vi "init.vi"(8 "error in":errorcluster, 10 "TBM module configuration in":refnum<class "TBM module configuration.lvclass">, 11 "UI Reference runtime in":refnum<class "UI Reference runtime.lvclass">) -> (0 "error out":errorcluster, 1 "data allocations":T1, 2 "execution settings":T4, 3 "UI Reference runtime out":refnum<class "UI Reference runtime.lvclass">)   [LabVIEW 2015, in "UI Reference runtime.lvclass"]
doc: "Provides an interface for initializing a module at runtime. While this interface performs no operations, a child should provide an override which may open any necessary references or sessions, allocate necessary memory, and perform any final configuration validataion before providing the full configuration <b>execution data</b> to the calling process."
uses:
  UI Reference runtime.lvclass
  <vilib>/NI/Tag Bus Module Framework/module configuration/TBM module configuration.lvclass
  <vilib>/NI/Tag Bus Module Framework/runtime/execution settings.ctl
  <vilib>/NI/Tag Bus Module Framework/channel/data tables.ctl
  <vilib>/NI/Tag Bus/dictionary/data dictionary.lvclass
  <vilib>/NI/Tag Bus/dictionary table pair.ctl
  <vilib>/NI/Tag Bus/table/data table.ctl
  configuration/UI Reference configuration.lvclass
  UI Reference runtime.lvclass/UI Reference runtime.ctl
  <vilib>/NI/Tag Bus Module Framework/channel/TBM channel.lvclass
  <vilib>/NI/Tag Bus Module Framework/runtime/TBM module execution interface.lvclass
  <vilib>/NI/Tag Bus/tag bus.lvlib
  <vilib>/NI/Tag Bus/table/data table.lvlib
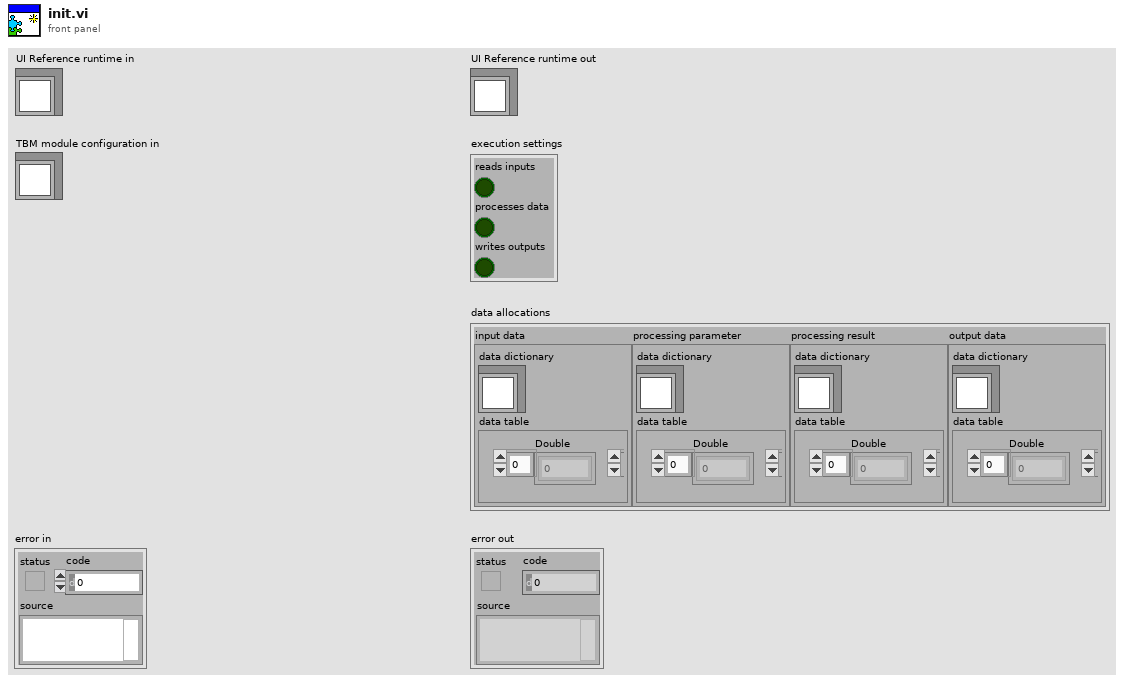
[diagram p1: front panel]
types:
  T1 = typedef "TBM channel.lvclass/data tables.ctl" = cluster{"input data":T2, "processing parameter":T2, "processing result":T2, "output data":T2}
  T2 = typedef "tag bus.lvlib/dictionary table pair.ctl" = cluster{"data dictionary":refnum<class "data dictionary.lvclass">, "data table":T3}
  T3 = typedef "tag bus.lvlib/data table.lvlib/data table.ctl" = cluster{"Double":dbl[], "Single":sgl[], "I64":i64[], "I32":i32[], "I16":i16[], "I8":i8[], "U64":u64[], "U32":u32[], "U16":u16[], "U8":u8[], "Boolean":bool[], "String":string[], "Array of Double":cluster{"DBL Array":dbl[]}[], "Array of Single":cluster{"SGL Array":sgl[]}[], "Array of I64":cluster{"I64 Array":i64[]}[], "Array of I32":cluster{"I32 Array":i32[]}[], "Array of I16":cluster{"I16 Array":i16[]}[], "Array of I8":cluster{"I8 Array":i8[]}[], "Array of U64":cluster{"U64 Array":u64[]}[], "Array of U32":cluster{"U32 Array":u32[]}[], "Array of U16":cluster{"U16 Array":u16[]}[], "Array of U8":cluster{"U8 Array":u8[]}[], "Array of Boolean":cluster{"Boolean Array":bool[]}[], "Array of String":cluster{"String Array":string[]}[]}
  T4 = typedef "TBM module execution interface.lvclass/execution settings.ctl" = cluster{"reads inputs":bool, "processes data":bool, "writes outputs":bool}
  T5 = typedef "UI Reference runtime.lvclass/Mapping.ctl" = cluster{"data type":T6, "control indexes":i32[], "data indexes":i32[]}
  T6 = typedef "tag bus.lvlib/tag descriptor.lvclass/Data Type.ctl" = enum16{"Double", "Single", "I64", "I32", "I16", "I8", "U64", "U32", "U16", "U8", "Boolean", "String", "Array of Double", "Array of Single", "Array of I64", "Array of I32", "Array of I16", "Array of I8", "Array of U64", "Array of U32", "Array of U16", "Array of U8", "Array of Boolean", "Array of String"}
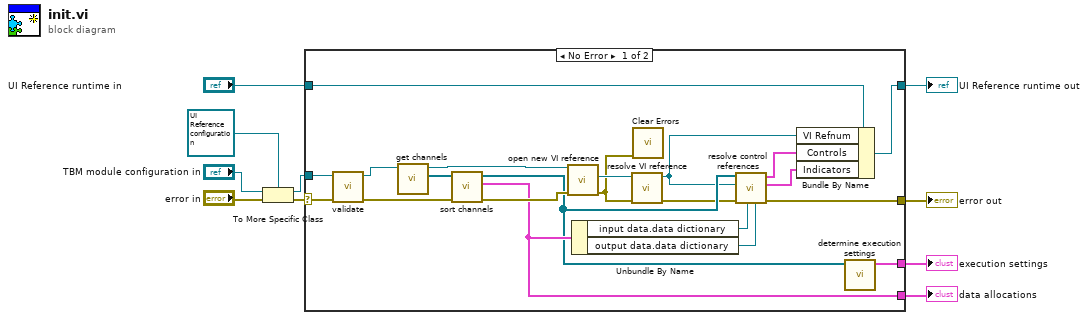
[diagram p0: block diagram]
diagram:
  n1 = To More Specific Class(target class=refnum<class "UI Reference configuration.lvclass"> refnum ("Synchronous module configuration"), reference="TBM module configuration in", error in="error in") -> (specific class reference=w9:refnum<class "UI Reference configuration.lvclass">, error out=w10:errorcluster)
  n2 = case shown="No Error" w10 {
    selector: w10 -> [w29 w32]
    tunnel: w9 -> [w28 _]
    tunnel: "UI Reference runtime in" -> [w17 w33]
    tunnel: [w16 w33] -> w4
    tunnel: [w11 w32] -> w3
    tunnel: [w21 _] -> w1
    tunnel: [w31 _] -> w2
    frame No Error {
      n3 = call-dynamic "validate.vi"("error in"=w29, "UI Reference configuration in"=w28) -> ("error out"=w30:errorcluster, "UI Reference configuration out"=w27:refnum<class "UI Reference configuration.lvclass">)  [unwired: 8 in]
      n4 = call-dynamic "get channels.vi"("UI Reference configuration in"=w27) -> ("channels"=w26:refnum<class "TBM channel.lvclass">[], "UI Reference configuration out"=w25:refnum<class "UI Reference configuration.lvclass">)  [unwired: 9 in]
      n5 = call <vilib>:"sort channels.vi"("error in"=w30, "channels in"=w26) -> ("error out"=w24:errorcluster, "data allocations"=w21:T1, "channels out"=w20:refnum<class "TBM channel.lvclass">[])  [unwired: 7 in]
      n6 = call "open new VI reference.vi"("error in"=w24, "UI Reference configuration in"=w25) -> ("error out"=w22:errorcluster, "VI Refnum"=w23:refnum<vi>)  [unwired: 7 in, 1 out]
      n7 = Unbundle By Name(w21) -> ("input data.data dictionary"=w19:refnum<class "data dictionary.lvclass">, "output data.data dictionary"=w18:refnum<class "data dictionary.lvclass">)
      n8 = call "resolve VI reference.vi"("error in"=w22, "VI reference"=w23) -> ("error out"=w14:errorcluster, "UI Ref"=w15:refnum<vi>)  [unwired: 8 in]
      n9 = call <vilib>:"Clear Errors.vi"("error in (no error)"=w22) -> ()  [unwired: 5 in, 2 out]
      n10 = call "resolve control references.vi"("output dictionary"=w18, "input dictionary"=w19, "error in"=w14, "UI Ref"=w15, "channels in"=w20) -> ("error out"=w11:errorcluster, "indicators"=w12:T5[], "controls"=w13:T5[])  [unwired: 4 in]
      n11 = Bundle By Name(cluster=w17, "VI Refnum"=w15, "Controls"=w13, "Indicators"=w12) -> (w16:refnum<class "UI Reference runtime.lvclass">)
      n12 = call <vilib>:"determine execution settings.vi"("channels"=w20) -> ("execution settings"=w31:T4)  [unwired: 10 in]
    }
    frame Error {
    }
  }
  "error out" <- w3
  "UI Reference runtime out" <- w4
  "execution settings" <- w2
  "data allocations" <- w1
